vi "CompressionPT.vi"() -> ()   [LabVIEW 2018]
doc: "PNA-X Example."
uses:
  PNA-X.lvlib
panel:
  out "XY Graph":cluster{"X-Axis":dbl[], "Data":dbl[]}(graph)
  out "VISA Out":refnum<visa-resource-name>
  in  "VISA IN":refnum<visa-resource-name>
  out "error out":errorcluster
  in  "error in (no error)":errorcluster
  # "1. Select Instrument Source from the \"VISA IN\" drop down.\n2. Run vi"
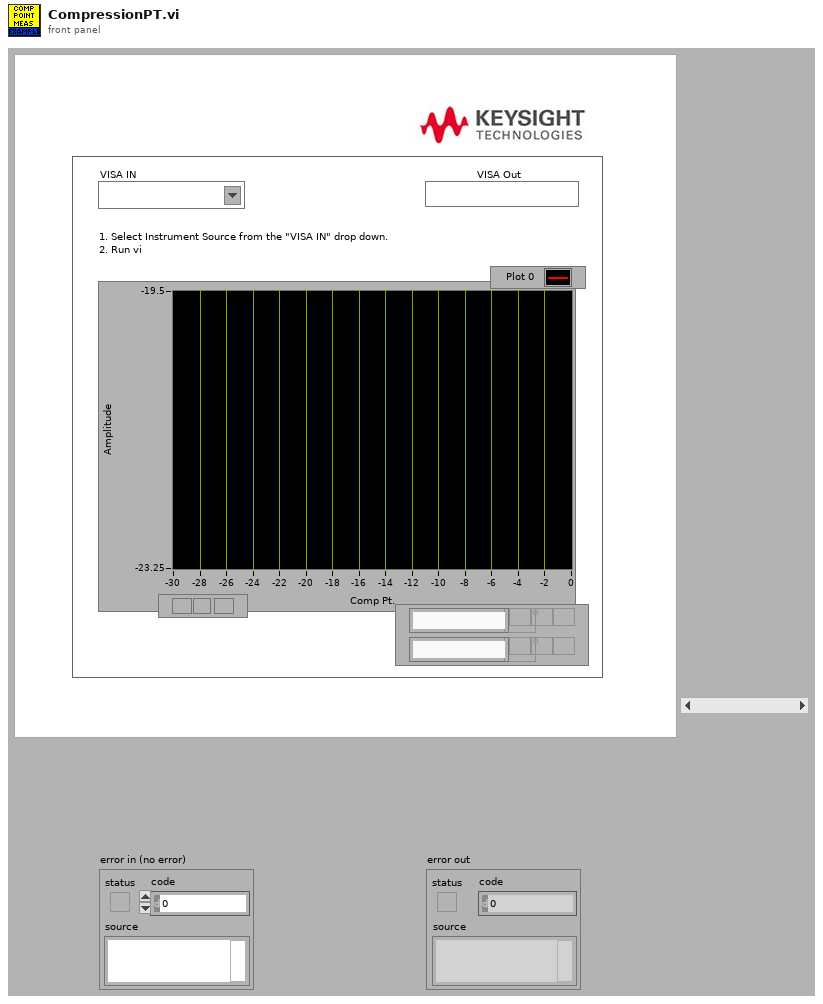
[diagram p1: front panel]
types:
  T1 = cluster{"Start Power":i32, "Stop Power":i32, "CW Frequency":dbl, "Format":string, "Compression Pt.":enum16{".1", ".3", "1", "3"}, "Average?":bool, "Avg. Factor":i32, "OK Button":bool}
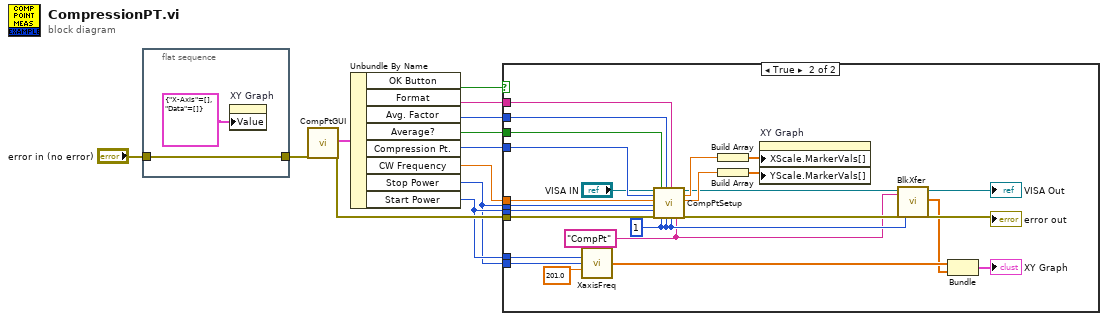
[diagram p0: block diagram]
diagram:
  n1 = flat-sequence {
    tunnel: "error in (no error)" -> [w13]
    tunnel: [w13] -> w1
    frame #0 {
      n2 = property on="XY Graph" class="XYGraph (strict)"("Value"=cluster{"X-Axis":dbl[], "Data":dbl[]} {"X-Axis"=[], "Data"=[]} ("XY Graph")) -> ()  [unwired: 2 in, 2 out]
    }
  }
  n3 = call "CompPtGUI.vi"("error in (no error)"=w1) -> ("output cluster"=w12:T1, "error out"=w5:errorcluster)  [unwired: 17 in]
  n4 = Unbundle By Name(w12) -> ("OK Button"=w11:bool, "Format"=w10:string, "Avg. Factor"=w9:i32, "Average?"=w8:bool, "Compression Pt."=w7:enum16{".1", ".3", "1", "3"}, "CW Frequency"=w6:dbl, "Stop Power"=w3:i32, "Start Power"=w4:i32)
  n5 = case shown="True" w11 {
    tunnel: w5 -> [_ w39]
    tunnel: w4 -> [_ w38]
    tunnel: w3 -> [_ w37]
    tunnel: w6 -> [_ w36]
    tunnel: w8 -> [_ w35]
    tunnel: w9 -> [_ w30]
    tunnel: w10 -> [_ w29]
    tunnel: w7 -> [_ w28]
    tunnel: w4 -> [_ w21]
    tunnel: w3 -> [_ w20]
    frame False {
    }
    frame True {
      w23 = "CompPt" ("Filename")
      w25 = 1 ("Channel")
      n6 = call "XaxisFreq.vi"("Start Frequency"=w21, "Stop Frequency"=w20, "Points"=201.0) -> ("X-Axis"=w19:dbl[])  [unwired: 12 in]
      n7 = call "CompPtSetup.vi"("VISA IN"="VISA IN", "Compression Pt."=w28, "CW Frq."=w36, "Stop Power"=w37, "Start Power"=w38, "error in"=w39, "AVG?"=w35, "Channel"=w25, "AVG"=w30, "Window"=w25, "Format"=w29, "Trace"=w25, "Filename"=w23) -> ("VISA Out"=w32:refnum<visa-resource-name>, "X Axis"=w34:dbl, "Y Real"=w33:dbl, "error out"=w31:errorcluster)  [unwired: 3 in]
      n8 = Build Array(w34) -> (w16:dbl[])
      n9 = Build Array(w33) -> (w15:dbl[])
      n10 = property on="XY Graph" class="XYGraph (strict)"("XScale.MarkerVals[]"=w16, "YScale.MarkerVals[]"=w15) -> ()  [unwired: 2 in, 2 out]
      n11 = call "BlkXfer.vi"("VISA IN"=w32, "FileName"=w23, "error in"=w31, "Channel"=w25) -> ("VISA Out"=→"VISA Out":refnum<visa-resource-name>, "Data"=w18:dbl[], "error out"=→"error out":errorcluster)  [unwired: 13 in]
      n12 = Bundle("X-Axis"=w19, "Data"=w18) -> (→"XY Graph":cluster{"X-Axis":dbl[], "Data":dbl[]})  [unwired: 1 in]
    }
  }
